vi "Enumeration.vi"(0 "read buffer":string, 5 "error in (no error)":errorcluster) -> (10 "Direccion 8":string, 11 "Direccion 6":string, 12 "Direccion 1":string, 13 "Direccion 5":string, 14 "Direccion 2":string, 15 "Direccion 7":string, 16 "Direccion 9":string, 17 "Direccion 3":string, 18 "Direccion 4":string, 19 "error out":errorcluster)   [LabVIEW 2021]
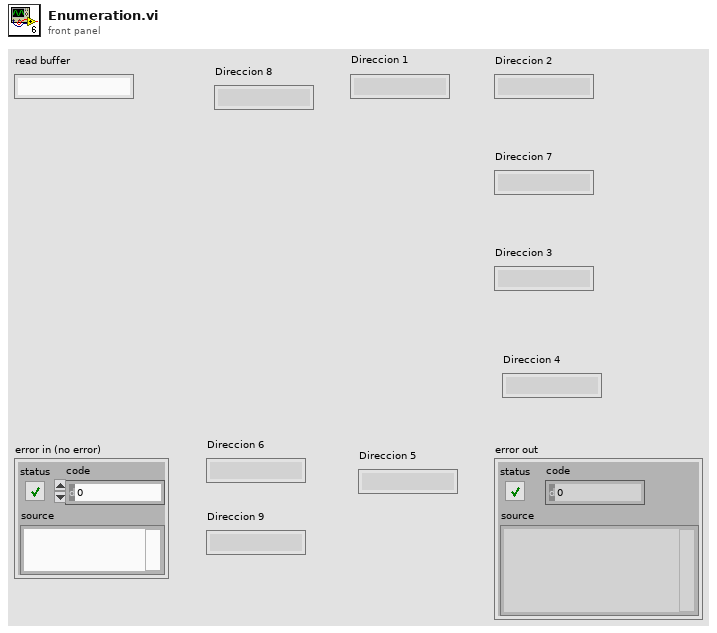
[diagram p1: front panel]
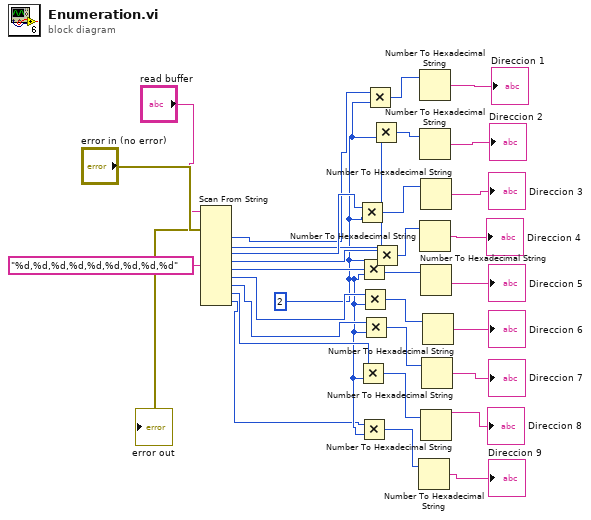
[diagram p0: block diagram]
diagram:
  w4 = 2
  n1 = Scan From String(format string="%d,%d,%d,%d,%d,%d,%d,%d,%d", input string="read buffer", error in="error in (no error)") -> (error out=→"error out":errorcluster, output 1=w9:i32, output 2=w10:i32, output 3=w11:i32, output 4=w12:i32, output 5=w13:i32, output 6=w14:i32, output 7=w15:i32, output 8=w6:i32, output 9=w1:i32)  [unwired: 10 in, 2 out]
  n2 = Multiply(x=w11, y=w4) -> (x*y=w18:i32)
  n3 = Multiply(x=w6, y=w4) -> (x*y=w23:i32)
  n4 = Multiply(x=w13, y=w4) -> (x*y=w20:i32)
  n5 = Multiply(x=w1, y=w4) -> (x*y=w3:i32)
  n6 = Multiply(x=w14, y=w4) -> (x*y=w21:i32)
  n7 = Multiply(x=w15, y=w4) -> (x*y=w22:i32)
  n8 = Multiply(x=w9, y=w4) -> (x*y=w16:i32)
  n9 = Multiply(x=w10, y=w4) -> (x*y=w17:i32)
  n10 = Multiply(x=w12, y=w4) -> (x*y=w19:i32)
  n11 = Number To Hexadecimal String(2:w3) -> (0:→"Direccion 9":string)  [unwired: 1 in]
  n12 = Number To Hexadecimal String(2:w16) -> (0:→"Direccion 1":string)  [unwired: 1 in]
  n13 = Number To Hexadecimal String(2:w17) -> (0:→"Direccion 2":string)  [unwired: 1 in]
  n14 = Number To Hexadecimal String(2:w19) -> (0:→"Direccion 4":string)  [unwired: 1 in]
  n15 = Number To Hexadecimal String(2:w18) -> (0:→"Direccion 3":string)  [unwired: 1 in]
  n16 = Number To Hexadecimal String(2:w20) -> (0:→"Direccion 5":string)  [unwired: 1 in]
  n17 = Number To Hexadecimal String(2:w23) -> (0:→"Direccion 8":string)  [unwired: 1 in]
  n18 = Number To Hexadecimal String(2:w22) -> (0:→"Direccion 7":string)  [unwired: 1 in]
  n19 = Number To Hexadecimal String(2:w21) -> (0:→"Direccion 6":string)  [unwired: 1 in]
